vi "GetMotorType.vi"(0 "CmdLib In":refnum<k24>, 5 "DeviceKey In":string, 7 "Device Address In":i32, 9 "Motor":i32, 11 "error in (no error)":errorcluster) -> (4 "CmdLib Out":refnum<k24>, 6 "DeviceKey Out":string, 8 "Device Address Out":i32, 10 "Motor Type":i32(ring) items=["NoMotor", "Undefined", "Tiny", "Standard"], 15 "error out":errorcluster)   [LabVIEW 2009]
uses:
  C:/Code/Apps/Utilities/Picomotor/PicomotorApp/Install/Samples/LabVIEW/Model 8742/LabVIEW 2009/CmdLib.dll
panel:
  in  "type":i32(ring) items=["NoMotor", "Undefined", "Tiny", "Standard"]
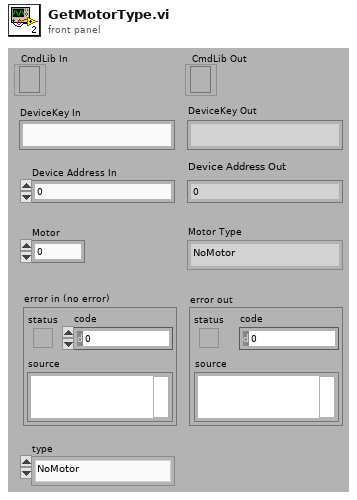
[diagram p1: front panel]
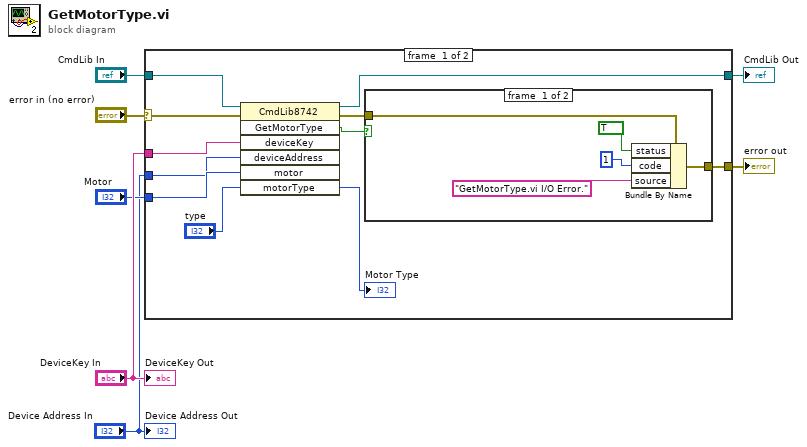
[diagram p0: block diagram]
diagram:
  n1 = case shown="No Error" "error in (no error)" {
    selector: "error in (no error)" -> [w15 w25]
    tunnel: "CmdLib In" -> [w18 w26]
    tunnel: [w17 w26] -> w6
    tunnel: "Motor" -> [w9 _]
    tunnel: "DeviceKey In" -> [w16 _]
    tunnel: [w12 w25] -> w3
    tunnel: "Device Address In" -> [w8 _]
    frame #0 {
      n2 = invoke class="CmdLib8742" method="GetMotorType"(reference=w18, error in=w15, "deviceKey"=w16, "deviceAddress"=w8, "motor"=w9, "motorType"="type") -> (reference out=w17:refnum<k24>, error out=w13:errorcluster, "GetMotorType"=w14:bool, "motorType"=→"Motor Type":i32)  [unwired: 1 in, 3 out]
      n3 = case shown="False" w14 {
        tunnel: w13 -> [w23 w24]
        tunnel: [w22 w24] -> w12
        frame #0 {
          n4 = Bundle By Name(cluster=w23, "status"=TRUE, "code"=1, "source"="GetMotorType.vi I/O Error.") -> (w22:errorcluster)
        }
        frame #1 {
        }
      }
    }
    frame #1 {
    }
  }
  "error out" <- w3
  "CmdLib Out" <- w6
  "DeviceKey Out" <- "DeviceKey In"
  "Device Address Out" <- "Device Address In"
